vi "Autonomous Mobile Robots.vi"(4 "Direction":bool=TRUE, 5 "Brake":bool=TRUE, 6 "Steering":dbl(slide) min=-1.0 max=1.0 step=1e-05 scale=-1.0..1.0) -> (0 "error out":errorcluster, 1 "fps":dbl, 2 "Map":picture, 3 "Camera":picture)   [LabVIEW 2025]
doc: "Enables users to control the vehicle's steering, throttle, brakes, starting position, and weather simulation in real time.\n\n*This is a free driving scenario with other vehicles spawning on specified positions in autopilot mode*"
panel:
  in  "Vehicle Start Position":i32=1 min=-1 max=2 step=1
  in  "stop":bool
  out "Weather Profiles":T1(array[cluster])
  # "Steering"
  # "Apply Brakes"
  # "Direction"
  # "FPS"
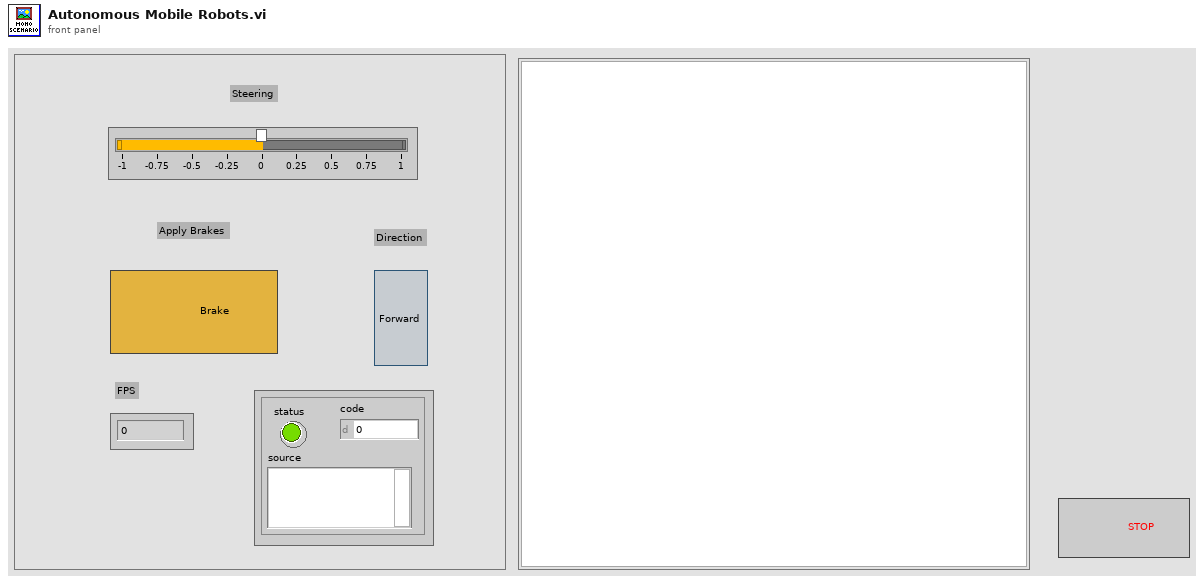
[diagram p1: front panel]
types:
  T1 = cluster{"id":string, "CloudColor":cluster{"A":sgl, "B":sgl, "G":sgl, "R":sgl}, "CloudOpacity":sgl, "Day":sgl, "FogCutoffDistance":sgl, "FogDensity":sgl, "FogHeightFalloff":sgl, "FogInscatteringColor":cluster{"A":sgl, "B":sgl, "G":sgl, "R":sgl}, "FogMaxOpacity":sgl, "FogStartDistance":sgl, "HorizonColor":cluster{"A":sgl, "B":sgl, "G":sgl, "R":sgl}, "HorizonFalloff":sgl, "Hours":sgl, "IsDaylightSavingTime":bool, "Latitude":sgl, "Longitude":sgl, "Minutes":sgl, "Month":sgl, "NorthOffset":sgl, "OverallSkyColor":cluster{"A":sgl, "B":sgl, "G":sgl, "R":sgl}, "OverideTimeBasedSunAngle":bool, "PrecipitationAccumulation":sgl, "PrecipitationAmount":sgl, "PrecipitationType":string, "SecondFogDensity":sgl, "SecondFogHeightFalloff":sgl, "SecondFogHeightOffset":sgl, "Seconds":sgl, "SkyLightColor":cluster{"A":sgl, "B":sgl, "G":sgl, "R":sgl}, "SkyLightIntensity":sgl, "StarBrightness":sgl, "SunAzimuthAngle":sgl, "SunBrightness":sgl, "SunDirectionalLightColor":cluster{"A":sgl, "B":sgl, "G":sgl, "R":sgl}, "SunDirectionalLightIntensity":sgl, "SunPolarAngle":sgl, "TimeZone":sgl, "WindAngle":sgl, "WindIntensity":sgl, "Year":sgl, "ZenithColor":cluster{"A":sgl, "B":sgl, "G":sgl, "R":sgl}, "bPrecipitation":bool, "bWind":bool}[]
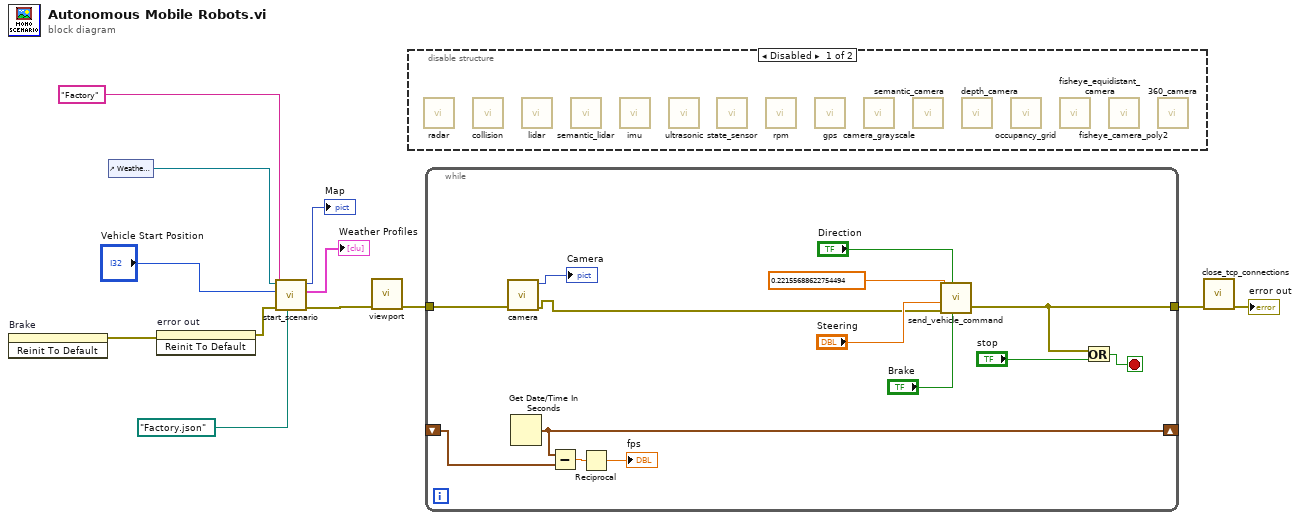
[diagram p0: block diagram]
diagram:
  n1 = invoke on="Brake" class="Bool (strict)" method="Reinit To Default"() -> (error out=w2:errorcluster)  [unwired: 3 in, 2 out]
  n2 = control-ref of="Weather Profiles"() -> (w1:refnum<vi>)
  n3 = invoke on="error out" class="Clust (strict)" method="Reinit To Default"(error in=w2) -> (error out=w12:errorcluster)  [unwired: 2 in, 2 out]
  n4 = call "start_scenario.vi"("Scenario Configuration"=path "Factory.json", "error in"=w12, "Select a map"="Factory", "Vehicle Start Position"="Vehicle Start Position", "Weather Profiles"=w1) -> ("error out"=w11:errorcluster, "Weather Profiles"=→"Weather Profiles":T1, "Map"=→"Map":picture)  [unwired: 2 in]
  n5 = call "viewport.vi"("Error In"=w11) -> ("Error Out"=w10:errorcluster)  [unwired: 6 in]
  n6 = disable-structure shown="Disabled" {
    frame Disabled {
      n7 = call "radar.vi"() -> ()  [unwired: 4 in, 5 out]
      n8 = call "collision.vi"() -> ()  [unwired: 4 in, 4 out]
      n9 = call "lidar.vi"() -> ()  [unwired: 4 in, 4 out]
      n10 = call "semantic_lidar.vi"() -> ()  [unwired: 4 in, 4 out]
      n11 = call "imu.vi"() -> ()  [unwired: 4 in, 4 out]
      n12 = call "ultrasonic.vi"() -> ()  [unwired: 3 in, 4 out]
      n13 = call "state_sensor.vi"() -> ()  [unwired: 4 in, 4 out]
      n14 = call "rpm.vi"() -> ()  [unwired: 4 in, 4 out]
      n15 = call "gps.vi"() -> ()  [unwired: 4 in, 4 out]
      n16 = call "camera_grayscale.vi"() -> ()  [unwired: 5 in, 5 out]
      n17 = call "semantic_camera.vi"() -> ()  [unwired: 5 in, 5 out]
      n18 = call "depth_camera.vi"() -> ()  [unwired: 5 in, 5 out]
      n19 = call "occupancy_grid.vi"() -> ()  [unwired: 5 in, 5 out]
      n20 = call "fisheye_equidistant_camera.vi"() -> ()  [unwired: 5 in, 4 out]
      n21 = call "fisheye_camera_poly2.vi"() -> ()  [unwired: 5 in, 4 out]
      n22 = call "360_camera.vi"() -> ()  [unwired: 5 in, 4 out]
    }
    frame Enabled {
    }
  }
  n23 = while {
    shift-right: [w26] -> _
    shift-left: _ -> [w25]
    tunnel: w10 -> [w14]
    tunnel: [w22] -> w8
    stop <- w23 stop-if-true
    n24 = call "camera.vi"("error In"=w14) -> ("Image"=→"Camera":picture, "error out"=w15:errorcluster)  [unwired: 4 in, 3 out]
    n25 = Get Date/Time In Seconds() -> (seconds since 1Jan1904=w26:timestamp)
    n26 = Subtract(x=w26, y=w25) -> (x-y=w24:dbl)
    n27 = Reciprocal(x=w24) -> (1/x=→"fps":dbl)
    n28 = call "send_vehicle_command.vi"("Brake"="Brake", "Drive mode"="Direction", "error in"=w15, "Right amount"="Steering", "Forward amount"=0.22155688622754494 ("Throttle")) -> ("error out"=w22:errorcluster)  [unwired: 2 in]
    n29 = Or(x=w22, y="stop") -> (x .or. y?=w23:bool)
  }
  n30 = call "close_tcp_connections.vi"("error in"=w8) -> ("error out"=→"error out":errorcluster)  [unwired: 6 in]
